vi "High g status display calculator.vi"(5 "Monitoring":T2, 7 "Recording":T2, 9 "Data ready":T2, 12 "retreiving data":bool) -> (8 "High G monitoring status":T1)   [LabVIEW 2011]
uses:
  Measurments Handling/Status Digitalish.ctl
  Stroker/High G staus list.ctl
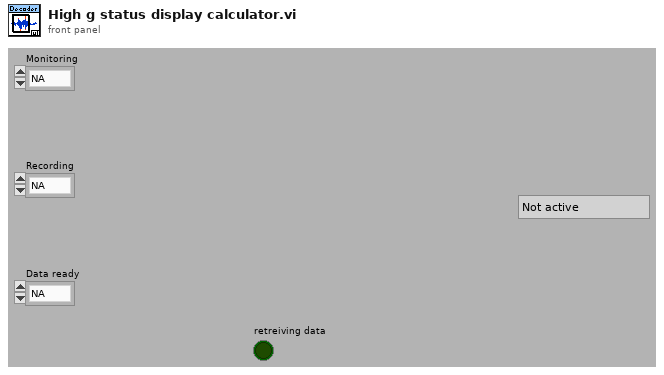
[diagram p1: front panel]
types:
  T1 = typedef "High G staus list.ctl" = enum16{"Not active", "Monitoring", "Recording", "Data ready", "Unknown", "Transferring data"}
  T2 = typedef "Status Digitalish.ctl" = enum16{"NA", "False", "True"}
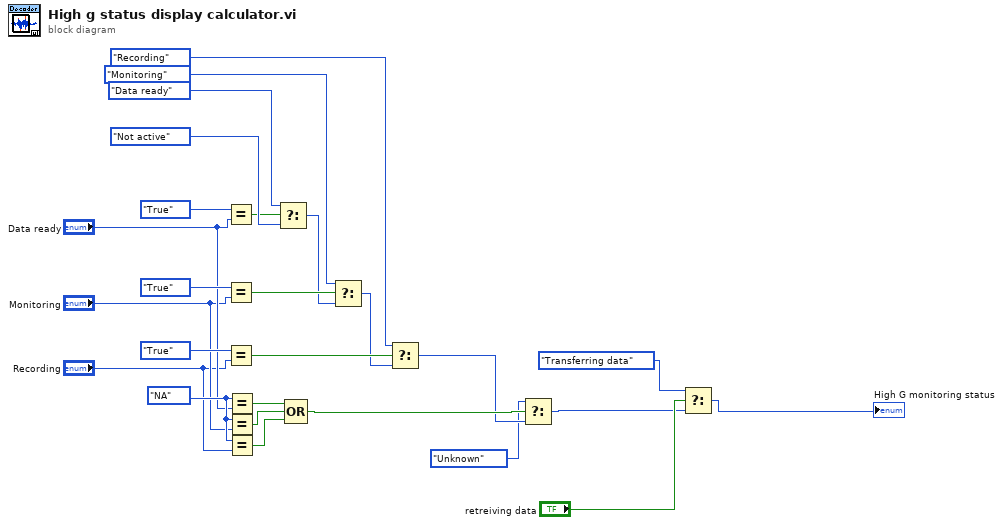
[diagram p0: block diagram]
diagram:
  w14 = Status_Digitalish."NA" ("x")
  n1 = Equal?(x=Status_Digitalish."True", y="Data ready") -> (x = y?=w21:bool)
  n2 = Equal?(x=Status_Digitalish."True", y="Monitoring") -> (x = y?=w20:bool)
  n3 = Equal?(x=Status_Digitalish."True", y="Recording") -> (x = y?=w17:bool)
  n4 = Equal?(x=w14, y="Data ready") -> (x = y?=w10:bool)
  n5 = Equal?(x=w14, y="Monitoring") -> (x = y?=w9:bool)
  n6 = Equal?(x=w14, y="Recording") -> (x = y?=w8:bool)
  n7 = Select(t=High_G_staus_list."Data ready", s=w21, f=High_G_staus_list."Not active" ("High G monitoring status")) -> (s? t:f=w19:T1)
  n8 = Compound Arithmetic op=OR(w10, w9, w8) -> (w7:bool)
  n9 = Select(t=High_G_staus_list."Monitoring", s=w20, f=w19) -> (s? t:f=w16:T1)
  n10 = Select(t=High_G_staus_list."Recording", s=w17, f=w16) -> (s? t:f=w6:T1)
  n11 = Select(t=High_G_staus_list."Unknown", s=w7, f=w6) -> (s? t:f=w3:T1)
  n12 = Select(t=High_G_staus_list."Transferring data", s="retreiving data", f=w3) -> (s? t:f=→"High G monitoring status":T1)
